vi "ClearTrigger.vi"(11 "错误输入（无错误）":errorcluster) -> (3 "错误输出":errorcluster)   [LabVIEW 2016]
uses:
  PLC-Lab/lib/gusb.dll
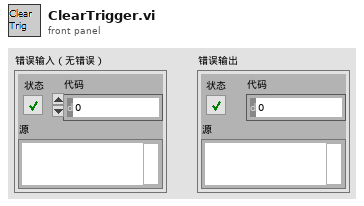
[diagram p1: front panel]
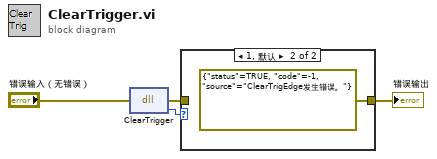
[diagram p0: block diagram]
diagram:
  n1 = dll-call lib="E:/Camproject/2018/2018.1Labview/PLC-Lab/lib/gusb.dll" fn="ClearTrigger"(error in="错误输入（无错误）") -> (error out=w2:errorcluster, "返回类型"=w3:i32)  [unwired: 2 in, 1 out]
  n2 = case shown="1, 默认" w3 {
    tunnel: w2 -> [w5 _]
    tunnel: [w5 errorcluster {"status"=TRUE, "code"=-1, "source"="ClearTrigEdge发生错误。"} ("错误常量")] -> w1
    frame 0 {
    }
    frame 1, Default {
    }
  }
  "错误输出" <- w1
